vi "PH_Cont-601k_PSU.PC R2S.vi"(0 "VI in":refnum<vi>, 2 "R2S":bool, 5 "error in (no error)":errorcluster) -> (14 "VI out":refnum<vi>, 17 "\"R2S\" changed":bool, 19 "error out":errorcluster)   [LabVIEW 2014, in "PH_Cont-601k_PSU.lvlib"]
uses:
  PH_Cont-601k_PSU.lvlib
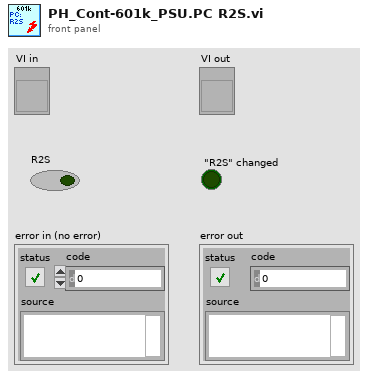
[diagram p1: front panel]
types:
  T1 = typedef "PH_Cont-601k_PSU.lvlib/PH_Cont-601k_PSU.i attribute.ctl" = cluster{"GUI Refs":T2, "Interlock":bool, "Service ID applied Voltage":i32, "Device Settings":cluster{"Configuration":T3, "Flash Interval [s]":dbl, "Mode":T4, "Voltage [V]":u16, "Charge":bool, "VISA resource name":refnum<visa-resource-name>}, "Readyness":T5, "Information":cluster{"VISA resource name":refnum<visa-resource-name>, "Tagname Power On":string, "Interlock":cluster{"Instance":string, "Tagname":string}, "Limits [V]":cluster{"Lower":dbl, "Upper":dbl}, "Tagname PSU On":string}, "R2S":bool, "Charge is allowed":bool}
  T2 = typedef "PH_Cont-601k_PSU.lvlib/PH_Cont-601k_PSU.GUI Refs.ctl" = cluster{"Power On":refnum<vi>, "Hard- and Software":refnum<vi>, "Device Status":refnum<vi>, "Device Error":refnum<vi>, "Configuration":refnum<vi>, "Flash Interval [s]":refnum<vi>, "Interlock":refnum<vi>, "Interlock Indicator":refnum<vi>, "Voltage [V]":refnum<vi>, "Readyness":refnum<vi>, "Mode":refnum<vi>, "Reset Error":refnum<vi>, "Expert working":refnum<vi>, "Charge":refnum<vi>, "PSU On":refnum<vi>}
  T3 = typedef "PH_Cont-601k_PSU.lvlib/PH_Cont-601k_PSU.Configuration.ctl" = u16
  T4 = typedef "PH_Cont-601k_PSU.lvlib/PH_Cont-601k_PSU.Mode.ctl" = enum32{"STOP", "STANDBY", "READY", "EMISSION", "ERROR"}
  T5 = typedef "PH_Cont-601k_PSU.lvlib/PH_Cont-601k_PSU.Readyness.ctl" = cluster{"Program":T6, "Device":T7}
  T6 = typedef "PH_Cont-601k_PSU.lvlib/PH_Cont-601k_PSU.Readyness Program.ctl" = enum32{"OFF", "POWER", "INTERLOCK"}
  T7 = typedef "PH_Cont-601k_PSU.lvlib/PH_Cont-601k_PSU.Readyness Device.ctl" = enum32{"OFF", "CONNECTING", "CONNECTED", "OPERATING", "EOC", "ERROR"}
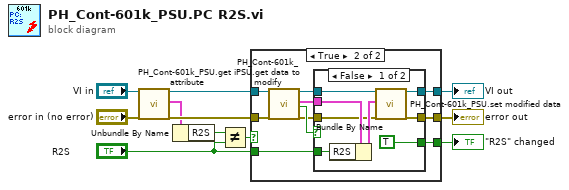
[diagram p0: block diagram]
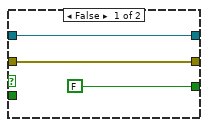
[diagram p2: hidden frame]
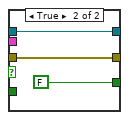
[diagram p3: hidden frame]
diagram:
  n1 = call "PH_Cont-601k_PSU.get i attribute.vi"("i ref in"="VI in", "error in (no error)"="error in (no error)") -> ("i ref out"=w6:refnum<vi>, "i attribute"=w5:T1, "error out"=w8:errorcluster)  [unwired: 15 in]
  n2 = Unbundle By Name(w5) -> ("R2S"=w4:bool)
  n3 = Not Equal?(x=w4, y="R2S") -> (x != y?=w3:bool)
  n4 = case shown="True" w3 {
    tunnel: [w13 w24] -> w11
    tunnel: [w14 w23] -> w10
    tunnel: w8 -> [w13 w18]
    tunnel: w6 -> [w14 w17]
    tunnel: "R2S" -> [_ w16]
    tunnel: [FALSE w15] -> w1
    frame False {
    }
    frame True {
      n5 = call "PH_Cont-601k_PSU.get data to modify.vi"("i ref in"=w17, "error in (no error)"=w18) -> ("i ref out"=w20:refnum<vi>, "i attribute"=w21:T1, "timed out"=w22:bool, "error out"=w19:errorcluster)  [unwired: 14 in]
      n6 = case shown="False" w22 {
        tunnel: [w28 w34] -> w24
        tunnel: w19 -> [w25 w34]
        tunnel: w20 -> [w32 w35]
        tunnel: [w29 w35] -> w23
        tunnel: w21 -> [w31 _]
        tunnel: w16 -> [w27 _]
        tunnel: [TRUE FALSE] -> w15
        frame False {
          n7 = Bundle By Name(cluster=w31, "R2S"=w27) -> (w30:T1)
          n8 = call "PH_Cont-601k_PSU.set modified data.vi"("i ref in"=w32, "i attribute"=w30, "error in (no error)"=w25) -> ("i ref out"=w29:refnum<vi>, "error out"=w28:errorcluster)  [unwired: 15 in]
        }
        frame True {
        }
      }
    }
  }
  "error out" <- w11
  "VI out" <- w10
  "\"R2S\" changed" <- w1
